vi "Datagridview Data.vi"(8 "Array":bool[](array[boolean]), 9 "data":string[][](array[string])) -> (3 "Array 3":T2(array[cluster]))   [LabVIEW 2013]
uses:
  Shared/LabVIEWdotNetDataGrid-master/source/GridColumn/ColumnType.ctl
  Shared/LabVIEWdotNetDataGrid-master/source/GridColumn/GridColumn.lvclass
panel:
  out "element":string
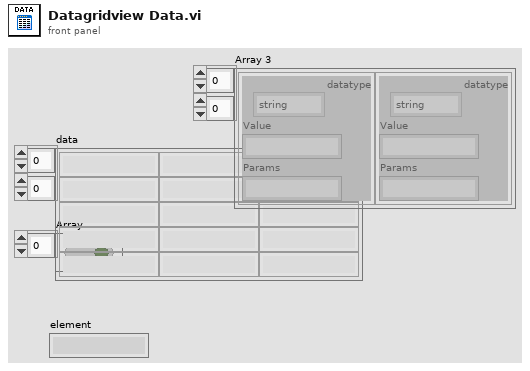
[diagram p1: front panel]
types:
  T1 = typedef "DataGrid.lvlib/GridColumn.lvclass/ColumnType.ctl" = enum16{"string", "image", "check", "numeric", "timestamp", "button", "combo", "link"}
  T2 = cluster{"datatype":T1, "Value":string, "Params":string}[][]
  T3 = typedef "mysql_authentication.ctl" = cluster{"User":string, "Password":string, "Database":string}
  T4 = cluster{"Port":u16, "IP Address":string, "Authentication":T3}
  T5 = cluster{"datatype":T1, "Value":string, "Params":string}
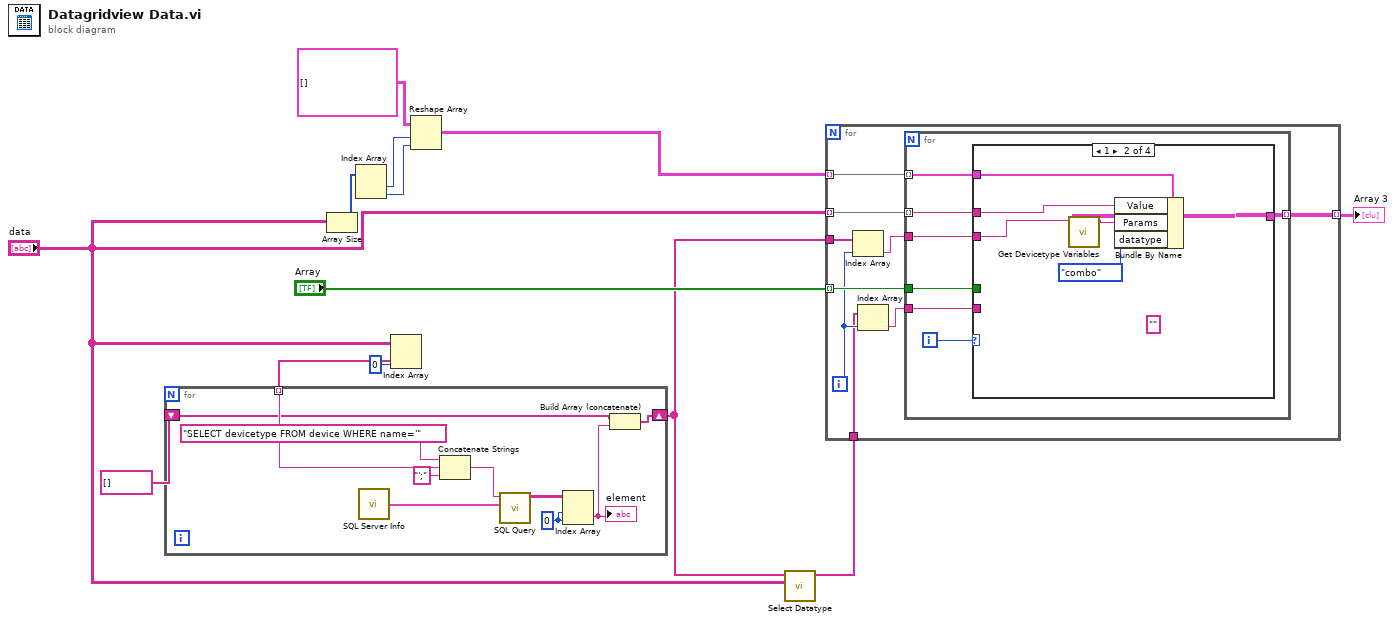
[diagram p0: block diagram]
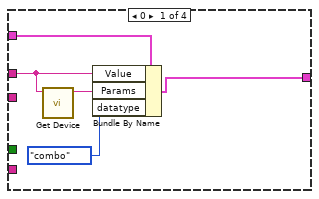
[diagram p2: hidden frame]
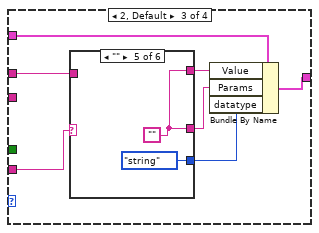
[diagram p3: hidden frame]
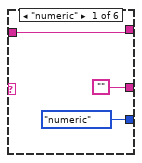
[diagram p4: hidden frame]
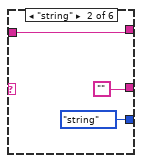
[diagram p5: hidden frame]
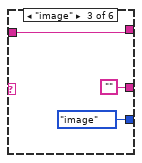
[diagram p6: hidden frame]
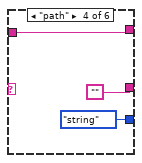
[diagram p7: hidden frame]
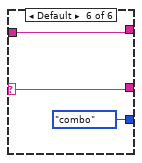
[diagram p8: hidden frame]
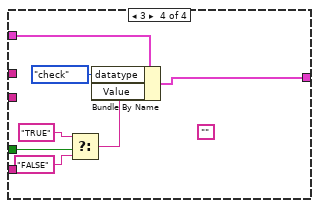
[diagram p9: hidden frame]
diagram:
  n1 = Array Size(array="data") -> (size(s)=w8:i32[])
  n2 = Index Array(array=w8) -> (element #1=w9:i32, element #2=w10:i32)  [unwired: 2 in]
  n3 = Index Array(array="data", index (col)=0 ("disabled index (col)")) -> (element=w5:string[])  [unwired: 1 in]
  n4 = for {
    tunnel: w5 -> [w18] mode=indexing
    shift-right: [w15] -> w2
    shift-left: string[] [] -> [w17]
    w19 = 0 ("disabled index (col)")
    n5 = call "SQL Server Info.vi"() -> ("SQL Server Info"=w14:T4)
    n6 = Concatenate Strings("SELECT devicetype FROM device WHERE name='", w18, "';" ("string")) -> (w21:string)
    n7 = call "SQL Query.vi"("SQL Server Info"=w14, "Query"=w21) -> ("data"=w20:string[][])  [unwired: 8 in, 1 out]
    n8 = Index Array(array=w20, index (row)=w19, index (col)=w19) -> (element=w16:string)
    "element" <- w16
    n9 = Build Array (concatenate)(w17, w16) -> (w15:string[])
  }
  n10 = Reshape Array(T2 [] ("Cells"), w9, w10) -> (w12:T2)
  n11 = call "Select Datatype.vi"("data"="data", "Devicetype"=w2) -> ("Datatype"=w3:string[])  [unwired: 9 in]
  n12 = for {
    tunnel: w12 -> [w32] mode=indexing
    tunnel: "data" -> [w30] mode=indexing
    tunnel: [w31] -> w11 mode=indexing
    tunnel: "Array" -> [w29] mode=indexing
    tunnel: w2 -> [w27]
    tunnel: w3 -> [w24]
    i -> [w26]
    n13 = Index Array(array=w27, index=w26) -> (element=w28:string)
    n14 = Index Array(array=w24, index=w26) -> (element=w25:string)
    n15 = for {
      tunnel: w32 -> [w38] mode=indexing
      tunnel: w30 -> [w36] mode=indexing
      tunnel: [w37] -> w31 mode=indexing
      tunnel: w28 -> [w35]
      tunnel: w29 -> [w34]
      tunnel: w25 -> [w33]
      i -> [w39]
      n16 = case shown="1" w39 {
        tunnel: w38 -> [w44 w50 w57 w81]
        tunnel: [w43 w49 w56 w79] -> w37
        tunnel: w36 -> [w41 w46 w51 _]
        tunnel: w35 -> [_ w45 _ _]
        tunnel: w34 -> [_ _ _ w78]
        tunnel: w33 -> [_ _ w53 _]
        frame 0 {
          n17 = call "Get Device.vi"("String"=w41) -> ("substring"=w40:string)  [unwired: 6 in, 2 out]
          n18 = Bundle By Name(cluster=w44, "Value"=w41, "Params"=w40, "datatype"=ColumnType."combo") -> (w43:T5)
        }
        frame 1 {
          (unwired) ""
          n19 = call "Get Devicetype Variables.vi"("string"=w45) -> ("substring"=w47:string)  [unwired: 8 in, 2 out]
          n20 = Bundle By Name(cluster=w50, "Value"=w46, "Params"=w47, "datatype"=ColumnType."combo") -> (w49:T5)
        }
        frame 2, Default {
          n21 = case shown="\"\"" w53 {
            selector: w53 -> [_ _ _ _ _ w73]
            tunnel: ["" "" "" "" w70 w73] -> w55
            tunnel: [ColumnType."numeric" ("datatype") ColumnType."string" ("datatype") ColumnType."image" ("datatype") ColumnType."string" ("datatype") ColumnType."string" ("datatype") ColumnType."combo" ("datatype")] -> w54
            tunnel: [w58 w61 w64 w67 w70 w72] -> w52
            tunnel: w51 -> [w58 w61 w64 w67 _ w72]
            frame "numeric" {
            }
            frame "string" {
            }
            frame "image" {
            }
            frame "path" {
            }
            frame "" {
              w70 = ""
            }
            frame Default {
            }
          }
          n22 = Bundle By Name(cluster=w57, "Value"=w52, "Params"=w55, "datatype"=w54) -> (w56:T5)
        }
        frame 3 {
          (unwired) ""
          n23 = Select(t="TRUE" ("element"), s=w78, f="FALSE" ("element")) -> (s? t:f=w76:string)
          n24 = Bundle By Name(cluster=w81, "datatype"=ColumnType."check", "Value"=w76) -> (w79:T5)
        }
      }
    }
  }
  "Array 3" <- w11
